vi "SimpleRamp_GeneratePoinNumber_v4.vi"(2 "error in (no error)":errorcluster, 3 "Error Locator":string, 4 "formula":string="sin(10*f)", 5 "Current Variable settings":T1[](array[typedef]), 6 "dt":dbl=1.0, 7 "Points":u32=10) -> (0 "error out":errorcluster, 1 "Suggested point number":u32=642)   [LabVIEW 2012]
doc: "This program evaluates an expression on a range and suggests an optimal number of points for that evaluation. It looks at the difference of the averave of points i and i+2 from point i+1, and has a front panel cap on that."
uses:
  TypeDefs/Active procedure variables.ctl
  <vilib>/Analysis/NI_AALBase.lvlib
panel:
  in  "Max Points":u32=65536
  in  "Max error tolarance":dbl=0.01 format="%#_6p"
  # "This computes the expression, where\n\"f\" on the domain [0,1]\nor\n\"t\" varaible is in absolute units."
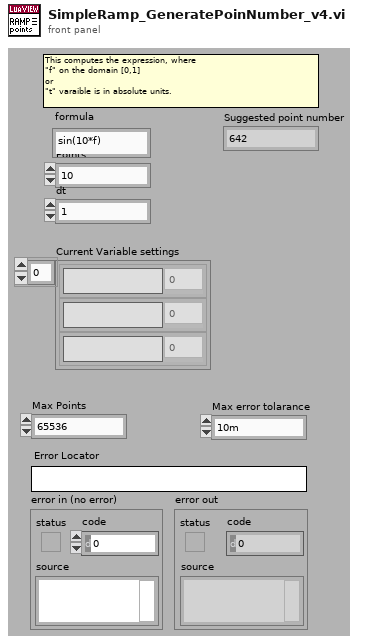
[diagram p1: front panel]
types:
  T1 = typedef "Active procedure variables.ctl" = cluster{"Procedure variable":string, "Value":dbl}
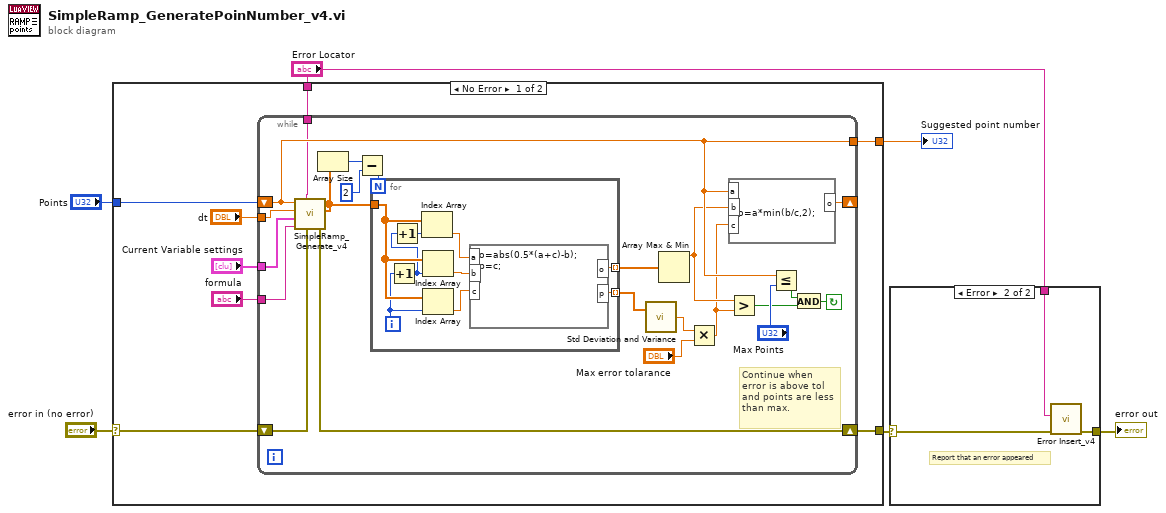
[diagram p0: block diagram]
diagram:
  n1 = case shown="No Error" "error in (no error)" {
    selector: "error in (no error)" -> [w11 w47]
    tunnel: [w10 w47] -> w3
    tunnel: [w8 w46] -> w4
    tunnel: "Points" -> [w9 w46]
    tunnel: "Error Locator" -> [w7 _]
    frame No Error {
      n2 = while {
        shift-right: [w24] -> _
        shift-left: w9 -> [w23]
        tunnel: "dt" -> [w36]
        tunnel: "Current Variable settings" -> [w35]
        tunnel: "formula" -> [w34]
        shift-right: [w32] -> w10
        shift-left: w11 -> [w33]
        tunnel: [w23] -> w8
        tunnel: w7 -> [w15]
        stop <- w27 continue-if-true
        # "Continue when \nerror is above tol\nand points are less\nthan max."
        n3 = call "SimpleRamp_Generate_v4.vi"("error in (no error)"=w33, "Error Locator"=w15, "formula"=w34, "Current Variable settings"=w35, "dt"=w36, "Points"=w23) -> ("error out"=w32:errorcluster, "y values"=w31:dbl[])  [unwired: 2 out]
        n4 = Array Size(array=w31) -> (size(s)=w20:i32)
        n5 = Subtract(x=w20, y=2) -> (x-y=w30:i32)
        n6 = for {
          N: w30 -> [_]
          tunnel: w31 -> [w45]
          tunnel: [w38] -> w29 mode=indexing
          tunnel: [w37] -> w19 mode=indexing
          i -> [w42]
          n7 = Increment(x=w42) -> (x+1=w43:i32)
          n8 = Increment(x=w43) -> (x+1=w44:i32)
          n9 = Index Array(array=w45, index=w44) -> (element=w41:dbl)
          n10 = Index Array(array=w45, index=w43) -> (element=w40:dbl)
          n11 = Index Array(array=w45, index=w42) -> (element=w39:dbl)
          n12 = formula code="o=abs(0.5*(a+c)-b);\np=c;"("a"=w41, "b"=w40, "c"=w39) -> ("o"=w38:dbl, "p"=w37:dbl)
        }
        n13 = call <vilib>:"Std Deviation and Variance.vi"("X"=w19) -> ("standard deviation"=w17:dbl)  [unwired: 1 in, 2 out]
        n14 = Array Max & Min(array=w29) -> (max value=w22:dbl)  [unwired: 3 out]
        n15 = Multiply(x=w17, y="Max error tolarance") -> (x*y=w16:dbl)
        n16 = formula code="o=a*min(b/c,2);"("a"=w23, "b"=w22, "c"=w16) -> ("o"=w24:dbl)
        n17 = Greater?(x=w22, y=w16) -> (0:w25:bool)
        n18 = Less Or Equal?(x=w23, y="Max Points") -> (x <= y?=w26:bool)
        n19 = And(x=w26, y=w25) -> (x .and. y?=w27:bool)
      }
    }
    frame Error {
    }
  }
  "Suggested point number" <- w4
  n20 = case shown="Error" w3 {
    selector: w3 -> [w48 w51]
    tunnel: [w48 w50] -> w2
    tunnel: "Error Locator" -> [_ w49]
    frame No Error {
    }
    frame Error {
      # "Report that an error appeared"
      n21 = call "Error Insert_v4.vi"("error in (no error)"=w51, "error message (\"\")"=w49) -> ("error out"=w50:errorcluster)  [unwired: 1 in, 6 out]
    }
  }
  "error out" <- w2
